vi "Grab Hatch Auto.vi"   [LabVIEW 2018]
uses:
  SubSystems/Hatch Panel Intake/Hatch Panel Intake Global.vi
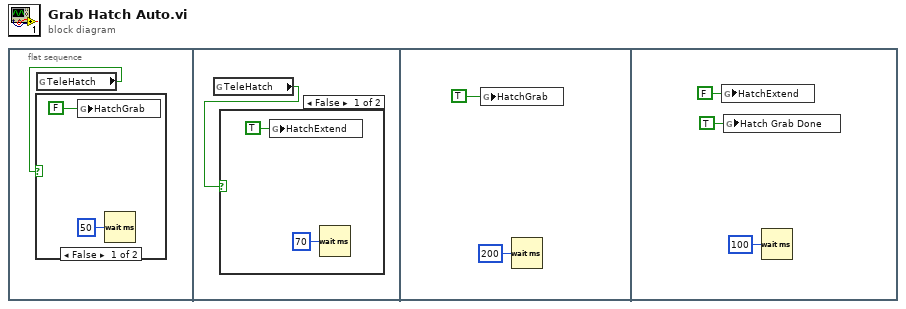
[diagram p0: block diagram]
diagram:
  n1 = flat-sequence {
    frame #0 {
      n2 = global read "Hatch Panel Intake Global.vi" "TeleHatch"() -> (w1:bool)
      n3 = case shown="False" w1 {
        frame False {
          n4 = global write "Hatch Panel Intake Global.vi" "HatchGrab"(FALSE ("HatchExtend")) -> ()
          n5 = Wait (ms)(milliseconds to wait=u32 50) -> ()  [unwired: 1 out]
        }
        frame True {
        }
      }
    }
    frame #1 {
      n6 = global read "Hatch Panel Intake Global.vi" "TeleHatch"() -> (w4:bool)
      n7 = case shown="False" w4 {
        frame False {
          n8 = global write "Hatch Panel Intake Global.vi" "HatchExtend"(TRUE ("HatchExtend")) -> ()
          n9 = Wait (ms)(milliseconds to wait=u32 70) -> ()  [unwired: 1 out]
        }
        frame True {
        }
      }
    }
    frame #2 {
      n10 = global write "Hatch Panel Intake Global.vi" "HatchGrab"(TRUE ("HatchExtend")) -> ()
      n11 = Wait (ms)(milliseconds to wait=u32 200) -> ()  [unwired: 1 out]
    }
    frame #3 {
      n12 = global write "Hatch Panel Intake Global.vi" "HatchExtend"(FALSE ("HatchExtend")) -> ()
      n13 = global write "Hatch Panel Intake Global.vi" "Hatch Grab Done"(TRUE ("Hatch Grab Done")) -> ()
      n14 = Wait (ms)(milliseconds to wait=u32 100) -> ()  [unwired: 1 out]
    }
  }
